vi "LIA Test CORDIC FPGA.vi"() -> ()   [LabVIEW 2017]
uses:
  <instrlib>/_niInstr/Streaming/v1/Common/Stream State.ctl
  <vilib>/Platform/TimedLoop/XDataNode/timing_clust.ctl
  <vilib>/Platform/TimedLoop/XDataNode/nitl_modes.ctl
  <vilib>/Platform/TimedLoop/XDataNode/wakeup.ctl
  <instrlib>/_niInstr/DSP/v1/Shared/Public/IQ Data.ctl
  <vilib>/rvi/FXPMathLib/FxpSinAndCos/subVIs/nifxpmath_SinAndCos_SimConfig.ctl
  <vilib>/rvi/IPIntegrationNode/IPINode_Typedef/niFpgaIPINodeSupportedFamilies.ctl
  <vilib>/rvi/Emulation/niFpgaSctlEmulationGetInTimedLoop.vi
  <vilib>/rvi/Emulation/niFpgaEmulationReportErrorSimple.vi
  <vilib>/rvi/Emulation/niFpgaGetClockAttributes.vi
  <vilib>/rvi/Emulation/niFpgaCriticalErrorInLSC.vi
  <vilib>/rvi/eio/common/nirviEmuTemplateMethod_errors.vi
  <instrlib>/_niInstr/Basic Elements/v1/FPGA/Private/Count Up U64.vi
  <vilib>/rvi/IPIntegrationNode/IPINode_Utilities/niFpgaIPINodeSimCore.vi
  <vilib>/rvi/FXPMathLib/FxpSinAndCos/simVIs/DllFxpSinAndCosTemp_sub.vi
  <vilib>/rvi/interface/RandomDataEmulation/niFpgaRandomDataHandleErrors.vi
  <instrlib>/_niInstr/DSP/v1/FPGA/Public/Sub VIs/Frequency Shift/Frequency Shift - 2 spc.vi
  <vilib>/Platform/TimedLoop/XDataNode/XDataNode.xnode
  <vilib>/eio/EIONode/EIONode.xnode
  <vilib>/rvi/FXPMathLib/FxpAdd/XNode/nifxpmath_Add.xnode
  <vilib>/rvi/XilinxIP/XIPIN_XNode/niFpgaXIPIN.xnode
  LIA CORDIC FPGA/CORDIC/xsim.dir/CORDIC_E0096FA8D1514E84B38CB4A6ADC5C7EA/xsimk_E0096FA8D1514E84B38CB4A6ADC5C7EA.dll
  <vilib>/rvi/IPIntegrationNode/IPINode_Xnode/niFpgaIPINode.xnode
  <vilib>/rvi/FXPMathLib/FxpSinAndCos/XNode/nifxpmath_SinAndCos.xnode
  LIA Test CORDIC FPGA/Complex Multiplier/xsim.dir/Complex_Multiplier_DCAD7DD88FD1460A918E1FD78EBF0FD6/xsimk_DCAD7DD88FD1460A918E1FD78EBF0FD6.dll
  <vilib>/rvi/FXPMathLib/FxpMul/XNode/nifxpmath_Multiplier.xnode
  <vilib>/rvi/DataTransferAndStorage/Container/XNode/niFpgaContainer.xnode
  <vilib>/rvi/interface/RandomDataEmulation/nirviRandomDataFpgaReadWriteTemplate.vi
  <instrlib>/_niInstr/DSP/v1/Xnodes/Public/Frequency Shift/niInstr DSP v1 Frequency Shift FPGA.xnode
  <vilib>/Platform/TimedLoop/XDataNode/XDNodeRunTimeDep.lvlib
  <instrlib>/_niInstr/DSP/v1/FPGA/niInstr DSP v1 FPGA.lvlib
  <instrlib>/_niInstr/DSP/v1/Shared/niInstr DSP v1 Shared.lvlib
  <instrlib>/_niInstr/Streaming/v1/FPGA/niInstr Streaming v1 FPGA.lvlib
  <instrlib>/_niInstr/Basic Elements/v1/FPGA/niInstr Basic Elements v1 FPGA.lvlib
  <vilib>/rvi/FXPMathLib/sim/FxpSim.dll
  <instrlib>/_niInstr/Streaming/v1/Common/niInstr Streaming v1 Common.lvlib
panel:
  in  "Xilinx Cordic":bool
  out "multiply rdi count 0":u64
  in  "samples route (None)":T1(ring)=enum."IDL-Frequency_Shift"
  out "FIFO Q rdi count 0":u64
  in  "phase delta (pi rad) 0":fxp<+/-,32,1> format="%.32g"
  in  "clear all counters (F) 0":bool
  out "IO Module\\InitDone":bool
  out "IO Module\\User Error":u32
  in  "IO Module\\User Command":u32
  in  "IO Module\\User Command Valid":bool
  out "IO Module\\User Command Ready":bool
  in  "IO Module\\User Command Arg 0":u32
  in  "IO Module\\User Command Arg 1":u32
  out "IO Module\\User Command Error":u16
  out "IO Module\\User Command Return":u32
  out "IO Module\\User Command Return Valid":bool
  in  "ao.reset 0":bool
  in  "ao.level 0":fxp<+/-,18,1>
  in  "ao.carrier 0":fxp<+/-,48,0>=0.010000000000001563
  in  "Select NCO? 0":bool
  in  "output sample rate 0":fxp<+,48,1>=1.0
  out "FIFO I rdi count 0":u64
  out "idl fs rdi count 0":u64
  out "stream.metadata 0":u64
  out "stream.samples transferred 0":u64
  out "stream.state 0":T2
  in  "stream.request state 0":T2
  in  "stream.num samples 0":u64
  in  "nco enable (T) 0":bool=TRUE
  in  "nco frequency 0":fxp<+/-,48,0>
  in  "reset (F) 0":bool
  in  "frequency shift 0":fxp<+/-,48,0> format="%#.48g"
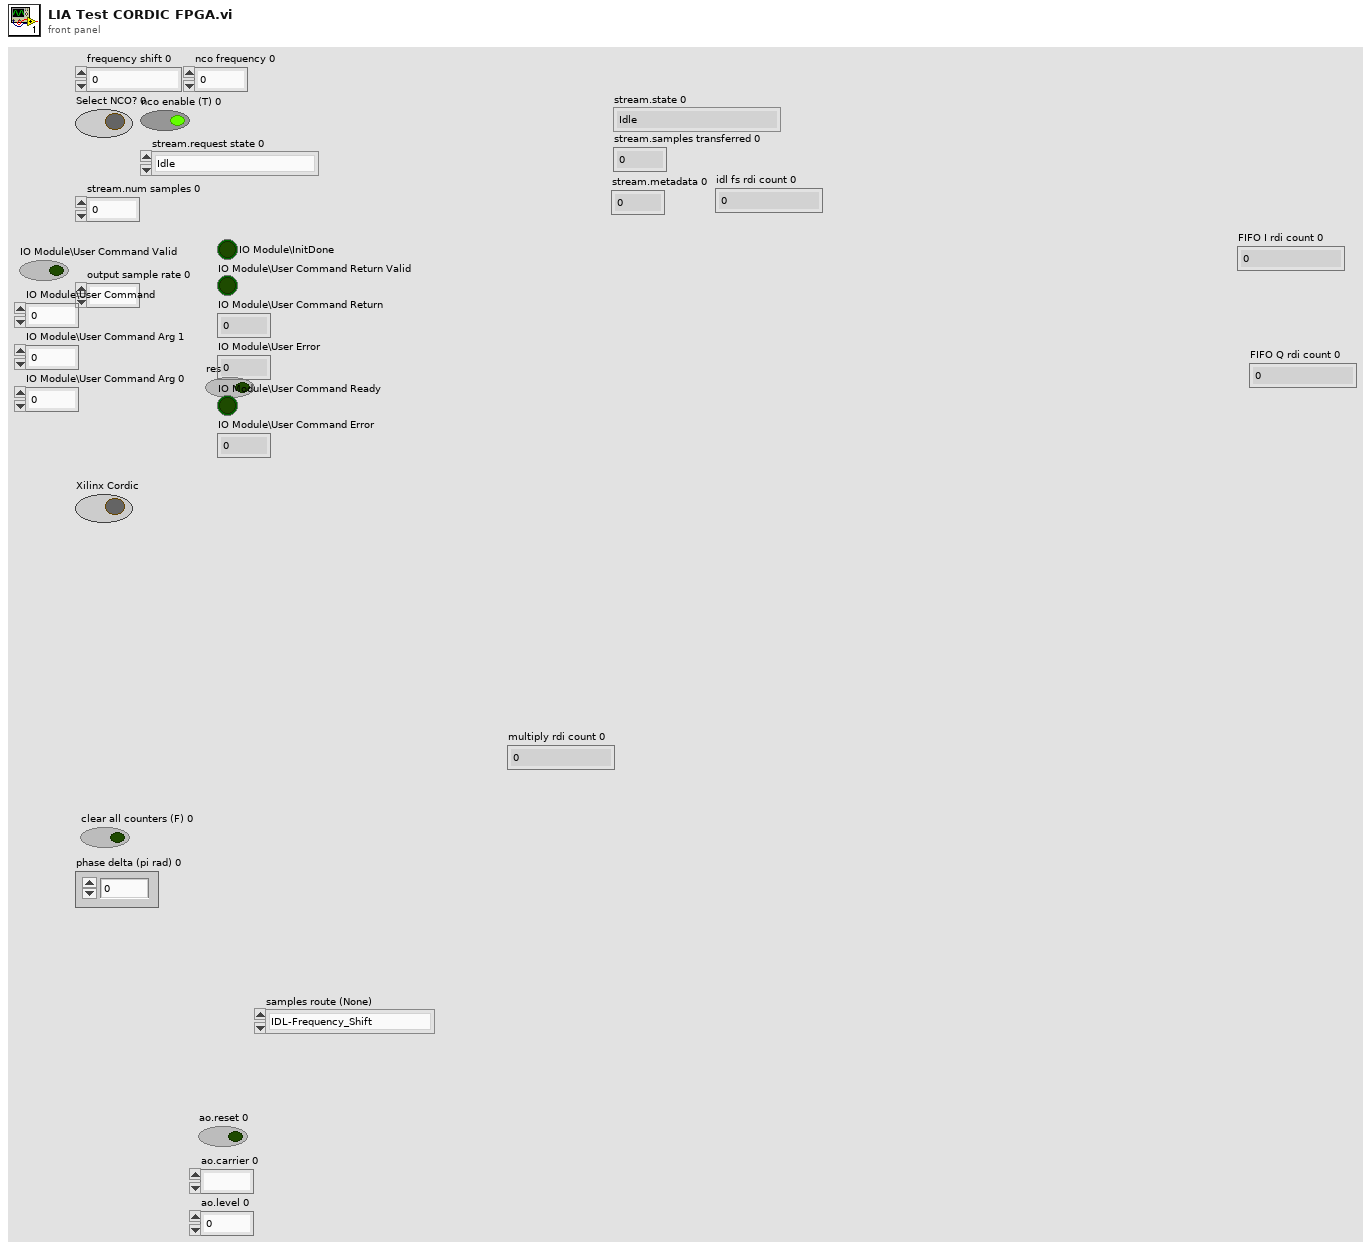
[diagram p1: front panel]
types:
  T1 = enum16{"None", "IDL-Frequency_Shift", "IDL-Frequency_Shift-FD", "CORDIC-Multiplication"}
  T2 = typedef "niInstr Streaming v1 Common.lvlib/Stream State.ctl" = enum8{"Idle", "Finite Transfer", "Continuous", "Done", "Error", "Not Ready", "Cancel"}
  T3 = typedef "XDNodeRunTimeDep.lvlib/timing_clust.ctl" = cluster{"Expected End [f-1]":u64, "Actual End [f-1]":u64, "Finished Late? [f-1]":bool, "Expected End [i-1]":u64, "Actual End [i-1]":u64, "Finished Late? [i-1]":bool, "Expected Start [i]":u64, "Actual Start [i]":u64, "Expected Start [f]":u64, "Actual Start [f]":u64, "Source Name":string, "Structure Name":string, "Period":i64, "Deadline":i64, "Offset":i64, "Start":i64, "Priority":i32, "Timeout":i32, "Mode":T4, "Wakeup Reason":T5, "Error":errorcluster, "Source Type":string, "Secondary Source Type":string, "Global End Time":u64, "Global Start Time":u64, "Frame Duration":u64, "Iteration Duration":u64, "Assigned CPU":i32, "I/O Scan Engine Mode":u32}
  T4 = typedef "XDNodeRunTimeDep.lvlib/nitl_modes.ctl" = enum32{"No Change", "Process missed periods, maintain original phase", "Discard missed periods, maintain original phase", "Process missed periods, ignore original phase", "Discard missed periods, ignore original phase"}
  T5 = typedef "XDNodeRunTimeDep.lvlib/wakeup.ctl" = enum32{"Normal", "Aborted", "Asynchronous wakeup", "Timing source error", "Timed loop error", "Timeout"}
  T6 = typedef "niInstr DSP v1 Shared.lvlib/IQ Data.ctl" = cluster{"I":fxp<+/-,18,1>, "Q":fxp<+/-,18,1>, "overflow":bool}
  T7 = typedef "niFpgaIPINodeSupportedFamilies.ctl" = cluster{"unlimited?":bool, "supported targets":string[]}
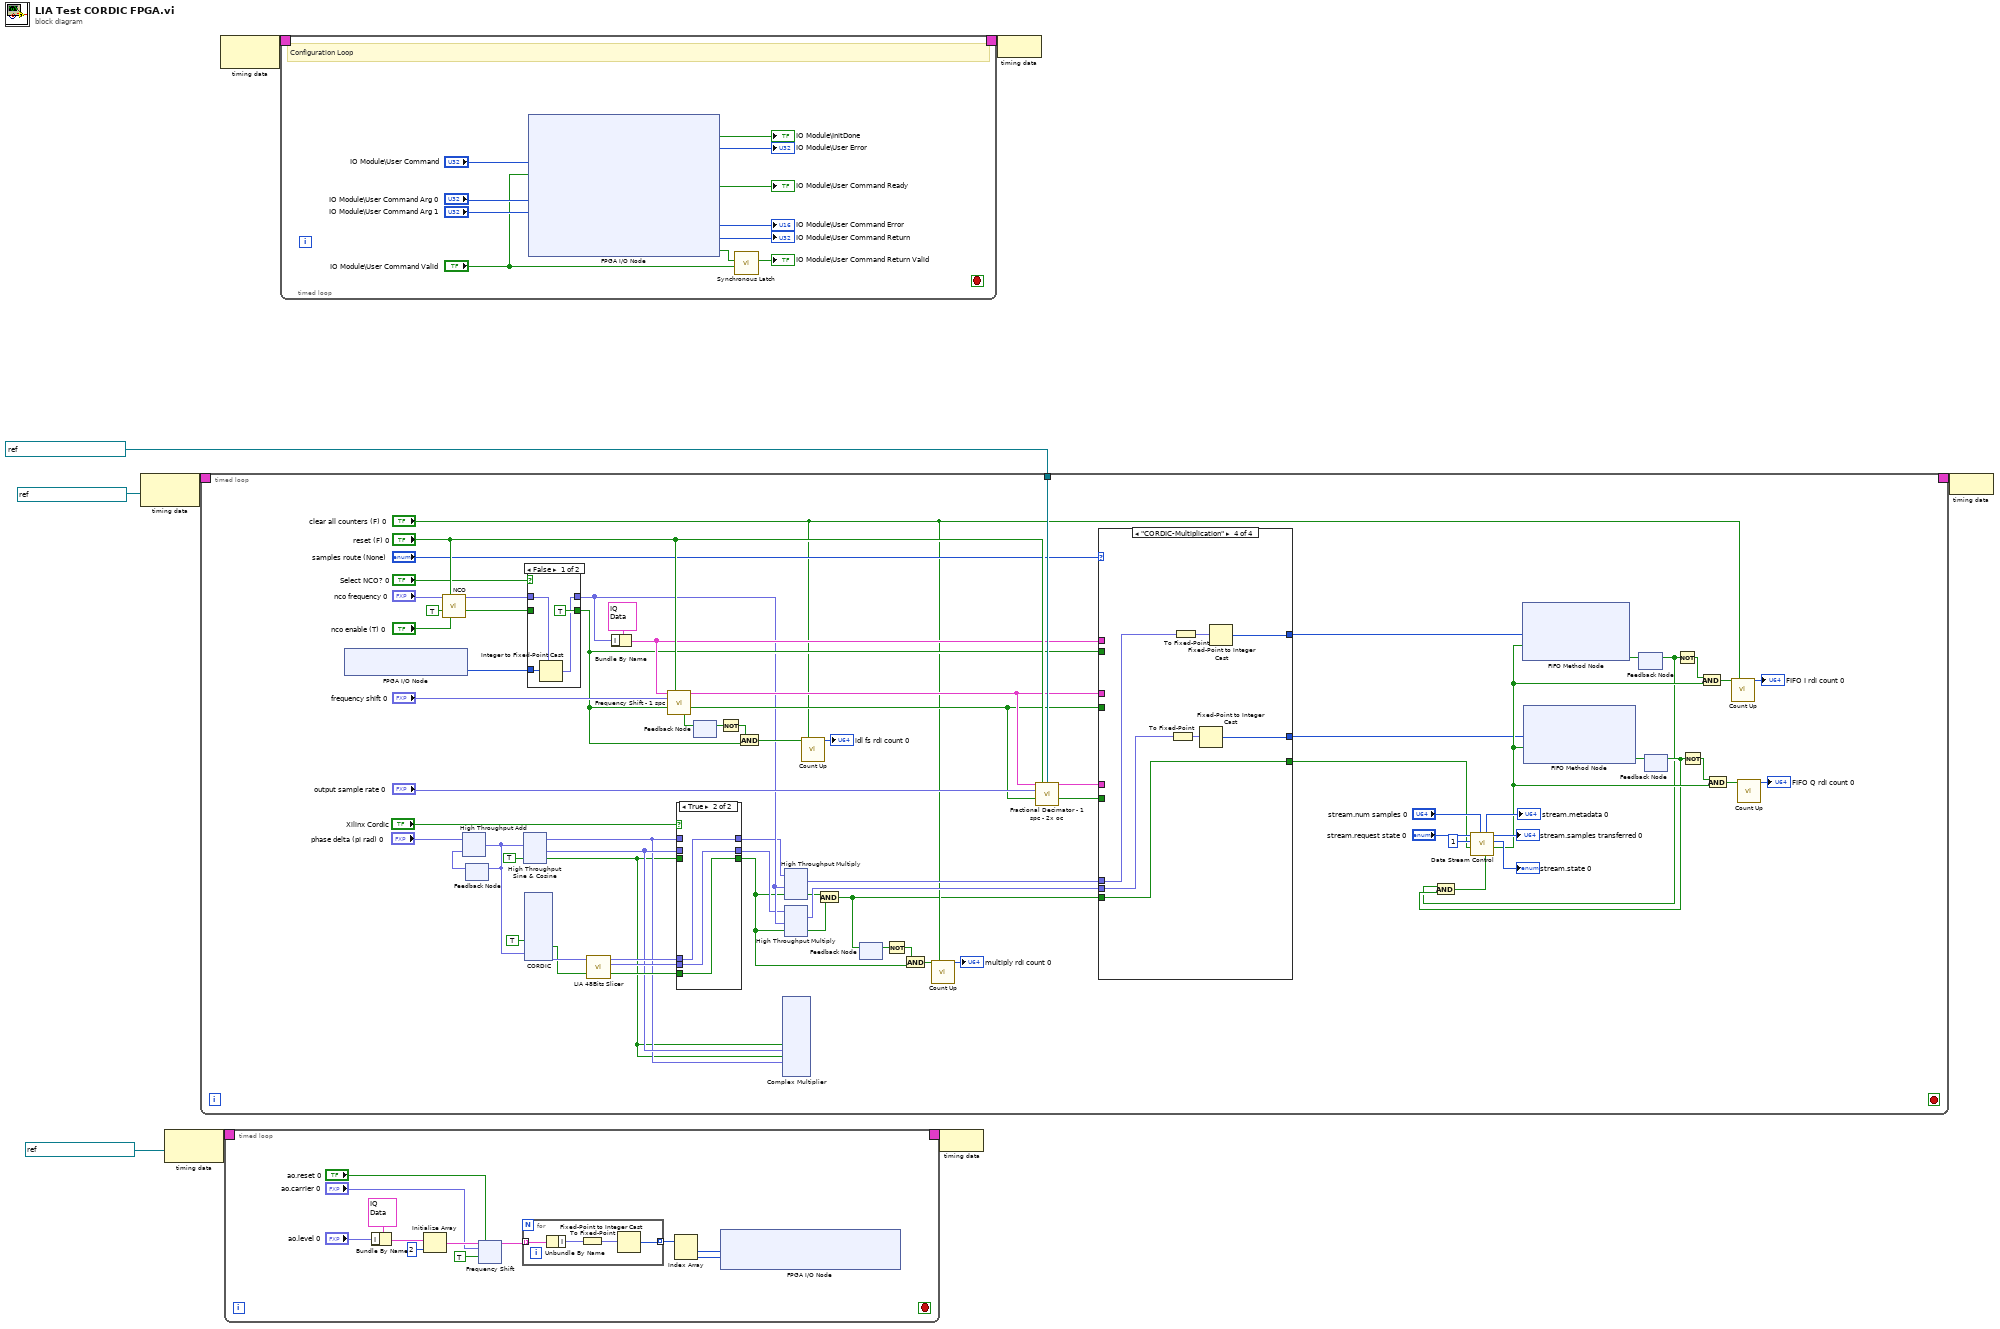
[diagram p0: block diagram]
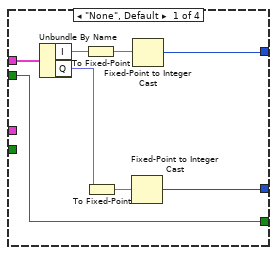
[diagram p4: hidden frame]
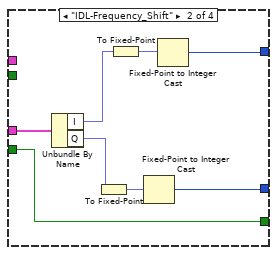
[diagram p5: hidden frame]
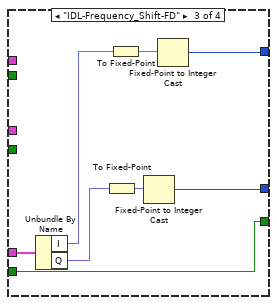
[diagram p6: hidden frame]
diagram:
  n1 = node-c288(refnum<k21> "IO Module\\Data Clock" ("Source Name")) -> (w9:T3)
  n2 = node-c288(refnum<k21> "IO Module\\Data Clock" ("Source Name")) -> (w5:T3)
  n3 = timed-loop {
    timing: w9 -> [_]
    timing-out: [_] -> w8
    tunnel: refnum<k21> "IO Module\\Data Clock 2x" ("clock x 2") -> [w61]
    stop <- _ stop-if-true
    n4 = xnode "FPGA I/O Node"() -> ("IO Module\\AI 0 Data N"=w38:i16)  [unwired: 1 in, 1 out]
    n5 = call <instrlib>:"NCO.vi"("frequency"="nco frequency 0", "reset"="reset (F) 0", "input valid"=TRUE, "enable (T)"="nco enable (T) 0") -> ("cosine out"=w41:fxp<+/-,18,1>, "output valid"=w39:bool)  [unwired: 9 in, 1 out]
    n6 = feedback #1() -> (w53:fxp<+/-,32,1>)  [unwired: 1 in]
    n7 = xnode ("High Throughput Add")("x"="phase delta (pi rad) 0", "y"=w53) -> ("x+y"=w26:fxp<+/-,32,1>)
    n8 = feedback-in #1(w26) -> ()
    n9 = xnode "High Throughput Sine & Cosine"("x (pi)"=w26, "input valid"=TRUE) -> ("sin(x)"=w11:fxp<+/-,22,2>, "cos(x)"=w12:fxp<+/-,22,2>, "output valid"=w10:bool)  [unwired: 1 in, 1 out]
    n10 = xnode ("CORDIC")("s_axis_phase_tvalid"=TRUE, "s_axis_phase_tdata"=w26) -> ("m_axis_dout_tvalid"=w14:bool, "m_axis_dout_tdata"=w19:fxp<+,48,48>)
    n11 = case shown="False" "Select NCO? 0" {
      tunnel: w41 -> [w211 w214]
      tunnel: [w209 w214] -> w24
      tunnel: [TRUE ("output valid") w213] -> w40
      tunnel: w39 -> [_ w213]
      tunnel: w38 -> [w212 _]
      frame False {
        n12 = Integer to Fixed-Point Cast(fixed-point type=w211, integer=w212) -> (fixed-point=w209:fxp<+/-,18,1>)
      }
      frame True {
      }
    }
    n13 = call "LIA 48Bits Slicer.vi"("m_axis_dout_tdata"=w19) -> ("Y"=w18:fxp<+/-,22,2>, "X"=w13:fxp<+/-,22,2>)  [unwired: 9 in]
    n14 = Bundle By Name(cluster=T6 {"I"=0.0, "Q"=0.0, "overflow"=FALSE} ("data in"), "I"=w24) -> (w43:T6)
    n15 = call <instrlib>:"Frequency Shift - 1 spc.vi"("data in"=w43, "reset"="reset (F) 0", "frequency shift"="frequency shift 0", "input valid"=w40) -> ("data out"=w52:T6, "output valid"=w37:bool, "ready for input"=w63:bool)  [unwired: 9 in]
    n16 = case shown="True" "Xilinx Cordic" {
      tunnel: [w148 w150] -> w22
      tunnel: w12 -> [w148 _]
      tunnel: [w147 w149] -> w21
      tunnel: w11 -> [w147 _]
      tunnel: [w146 w151] -> w20
      tunnel: w10 -> [w146 _]
      tunnel: w14 -> [_ w151]
      tunnel: w13 -> [_ w150]
      tunnel: w18 -> [_ w149]
      frame False {
      }
      frame True {
      }
    }
    n17 = feedback-in #2(w63) -> ()
    n18 = feedback #2() -> (w58:bool)  [unwired: 1 in]
    n19 = Not(x=w58) -> (.not. x?=w70:bool)
    n20 = And(x=w70, y=w40) -> (x .and. y?=w56:bool)
    n21 = xnode ("Complex Multiplier")("s_axis_a_tvalid"=w10, "s_axis_a_tdata"=w12, "s_axis_b_tvalid"=w10, "s_axis_b_tdata"=w11) -> ()  [unwired: 2 out]
    n22 = xnode ("High Throughput Multiply")("x"=w22, "y"=w24, "input valid"=w20) -> ("x*y"=w36:fxp<+/-,32,3>, "output valid"=w34:bool)  [unwired: 1 in, 1 out]
    n23 = xnode ("High Throughput Multiply")("x"=w21, "y"=w24, "input valid"=w20) -> ("x*y"=w35:fxp<+/-,32,3>, "output valid"=w33:bool)  [unwired: 1 in, 1 out]
    n24 = call-poly <instrlib>:"Count Up.vi"("increment"=w56, "reset"="clear all counters (F) 0") -> ("count out"=→"idl fs rdi count 0":u64)  [unwired: 13 in]
    n25 = And(x=w34, y=w33) -> (x .and. y?=w27:bool)
    n26 = feedback #3() -> (w31:bool)  [unwired: 1 in]
    n27 = feedback-in #3(w27) -> ()
    n28 = Not(x=w31) -> (.not. x?=w29:bool)
    n29 = And(x=w29, y=w20) -> (x .and. y?=w32:bool)
    n30 = call-poly <instrlib>:"Count Up.vi"("increment"=w32, "reset"="clear all counters (F) 0") -> ("count out"=→"multiply rdi count 0":u64)  [unwired: 13 in]
    n31 = call <instrlib>:"Fractional Decimator - 1 spc - 2x oc.vi"("data in"=w52, "reset"="reset (F) 0", "clock x 2"=w61, "output sample rate"="output sample rate 0", "input valid"=w37) -> ("data out"=w66:T6, "output valid"=w65:bool)  [unwired: 8 in, 1 out]
    n32 = case shown="\"CORDIC-Multiplication\"" "samples route (None)" {
      tunnel: w66 -> [_ _ w264 _]
      tunnel: w65 -> [_ _ w263 _]
      tunnel: w52 -> [_ w258 _ _]
      tunnel: [w247 w255 w263 w271] -> w64
      tunnel: [w249 w256 w265 w274] -> w46
      tunnel: [w248 w257 w266 w275] -> w45
      tunnel: w43 -> [w250 _ _ _]
      tunnel: w40 -> [w247 _ _ _]
      tunnel: w37 -> [_ w255 _ _]
      tunnel: w36 -> [_ _ _ w273]
      tunnel: w35 -> [_ _ _ w272]
      tunnel: w27 -> [_ _ _ w271]
      frame "None", Default {
        n33 = Unbundle By Name(w250) -> ("I"=w254:fxp<+/-,18,1>, "Q"=w252:fxp<+/-,18,1>)
        n34 = To Fixed-Point(number=w254) -> (fixed-point=w253:fxp<+/-,64,1>)  [unwired: 1 in]
        n35 = To Fixed-Point(number=w252) -> (fixed-point=w251:fxp<+/-,64,1>)  [unwired: 1 in]
        n36 = Fixed-Point to Integer Cast(1:w251) -> (0:w248:i64)
        n37 = Fixed-Point to Integer Cast(1:w253) -> (0:w249:i64)
      }
      frame "IDL-Frequency_Shift" {
        n38 = Unbundle By Name(w258) -> ("I"=w262:fxp<+/-,18,1>, "Q"=w260:fxp<+/-,18,1>)
        n39 = To Fixed-Point(number=w260) -> (fixed-point=w259:fxp<+/-,64,1>)  [unwired: 1 in]
        n40 = To Fixed-Point(number=w262) -> (fixed-point=w261:fxp<+/-,64,1>)  [unwired: 1 in]
        n41 = Fixed-Point to Integer Cast(1:w259) -> (0:w257:i64)
        n42 = Fixed-Point to Integer Cast(1:w261) -> (0:w256:i64)
      }
      frame "IDL-Frequency_Shift-FD" {
        n43 = Unbundle By Name(w264) -> ("I"=w270:fxp<+/-,18,1>, "Q"=w268:fxp<+/-,18,1>)
        n44 = To Fixed-Point(number=w268) -> (fixed-point=w267:fxp<+/-,64,1>)  [unwired: 1 in]
        n45 = To Fixed-Point(number=w270) -> (fixed-point=w269:fxp<+/-,64,1>)  [unwired: 1 in]
        n46 = Fixed-Point to Integer Cast(1:w267) -> (0:w266:i64)
        n47 = Fixed-Point to Integer Cast(1:w269) -> (0:w265:i64)
      }
      frame "CORDIC-Multiplication" {
        n48 = To Fixed-Point(number=w272) -> (fixed-point=w276:fxp<+/-,64,1>)  [unwired: 1 in]
        n49 = To Fixed-Point(number=w273) -> (fixed-point=w277:fxp<+/-,64,1>)  [unwired: 1 in]
        n50 = Fixed-Point to Integer Cast(1:w276) -> (0:w275:i64)
        n51 = Fixed-Point to Integer Cast(1:w277) -> (0:w274:i64)
      }
    }
    n52 = feedback #4() -> (w16:bool)  [unwired: 1 in]
    n53 = feedback #5() -> (w17:bool)  [unwired: 1 in]
    n54 = And(x=w16, y=w17) -> (x .and. y?=w15:bool)
    n55 = call <instrlib>:"Data Stream Control.vi"("ready for input?"=w15, "stream.num samples 0"="stream.num samples 0", "data valid"=w64, "element count"=u16 1, "stream.request state 0"="stream.request state 0") -> ("send data"=w47:bool, "stream.state 0"=→"stream.state 0":T2, "stream.samples transferred 0"=→"stream.samples transferred 0":u64, "stream.metadata 0"=→"stream.metadata 0":u64)  [unwired: 2 in, 1 out]
    n56 = xnode ("FIFO Method Node")("Element"=w46, "Input Valid"=w47) -> ("Ready for Input"=w60:bool)  [unwired: 1 in, 1 out]
    n57 = xnode ("FIFO Method Node")("Element"=w45, "Input Valid"=w47) -> ("Ready for Input"=w48:bool)  [unwired: 1 in, 1 out]
    n58 = feedback-in #4(w60) -> ()
    n59 = feedback-in #5(w48) -> ()
    n60 = Not(x=w16) -> (.not. x?=w59:bool)
    n61 = Not(x=w17) -> (.not. x?=w50:bool)
    n62 = And(x=w59, y=w47) -> (x .and. y?=w57:bool)
    n63 = And(x=w50, y=w47) -> (x .and. y?=w51:bool)
    n64 = call-poly <instrlib>:"Count Up.vi"("increment"=w57, "reset"="clear all counters (F) 0") -> ("count out"=→"FIFO I rdi count 0":u64)  [unwired: 13 in]
    n65 = call-poly <instrlib>:"Count Up.vi"("increment"=w51) -> ("count out"=→"FIFO Q rdi count 0":u64)  [unwired: 14 in]
  }
  n66 = node-c288() -> (w2:T3)  [unwired: 1 in]
  n67 = timed-loop {
    timing: w5 -> [_]
    timing-out: [_] -> w4
    stop <- _ stop-if-true
    n68 = Bundle By Name(cluster=T6 {"I"=0.0, "Q"=0.0, "overflow"=FALSE} ("output"), "I"="ao.level 0") -> (w287:T6)
    n69 = Initialize Array(w287, 2 ("dimension size")) -> (w291:T6[])
    n70 = xnode "Frequency Shift"("data in"=w291, "reset"="ao.reset 0", "frequency shift"="ao.carrier 0", "input valid"=TRUE) -> ("data out"=w283:T6[])  [unwired: 2 in, 2 out]
    n71 = for {
      tunnel: w283 -> [w294] mode=indexing
      tunnel: [w295] -> w282 mode=indexing
      n72 = Unbundle By Name(w294) -> ("I"=w293:fxp<+/-,18,1>)
      n73 = To Fixed-Point(number=w293) -> (fixed-point=w292:fxp<+/-,16,1>)  [unwired: 1 in]
      n74 = Fixed-Point to Integer Cast(1:w292) -> (0:w295:i16)
    }
    n75 = Index Array(array=w282) -> (element #1=w281:i16, element #2=w280:i16)  [unwired: 2 in]
    n76 = xnode "FPGA I/O Node"("IO Module\\AO 0 Data N-1 Data Clock"=w281, "IO Module\\AO 0 Data N Data Clock"=w280) -> ()  [unwired: 2 in, 2 out]
  }
  n77 = timed-loop {
    timing: w2 -> [_]
    timing-out: [_] -> w1
    stop <- _ stop-if-true
    # "Configuration Loop"
    n78 = xnode "FPGA I/O Node"("IO Module\\User Command"="IO Module\\User Command", "IO Module\\User Command Valid"="IO Module\\User Command Valid", "IO Module\\User Command Arg 0"="IO Module\\User Command Arg 0", "IO Module\\User Command Arg 1"="IO Module\\User Command Arg 1") -> ("IO Module\\InitDone"=→"IO Module\\InitDone":bool, "IO Module\\Clip Error Code"=→"IO Module\\User Error":u32, "IO Module\\User Command Ready"=→"IO Module\\User Command Ready":bool, "IO Module\\User Command Error"=→"IO Module\\User Command Error":u16, "IO Module\\User Command Return"=→"IO Module\\User Command Return":u32, "IO Module\\User Command Return Valid"=w308:bool)  [unwired: 10 in, 10 out]
    n79 = call <instrlib>:"Synchronous Latch.vi"("clear"="IO Module\\User Command Valid", "set"=w308) -> ("out"=→"IO Module\\User Command Return Valid":bool)  [unwired: 9 in]
  }
  n80 = node-c288(w4) -> ()
  n81 = node-c288(w1) -> ()
  n82 = node-c288(w8) -> ()
